vi "LogError.vi"(8 "error in (no error)":errorcluster, 10 "No Error":bool, 11 "Error Message":string) -> (0 "error out":errorcluster)   [LabVIEW 2017, in "Cls_AggHandler.xnode"]
uses:
  <vilib>/Utility/AggHandler/Cls_AggHandler.xnode
panel:
  out "Array":string[](array[string])
  in  "Clear":bool
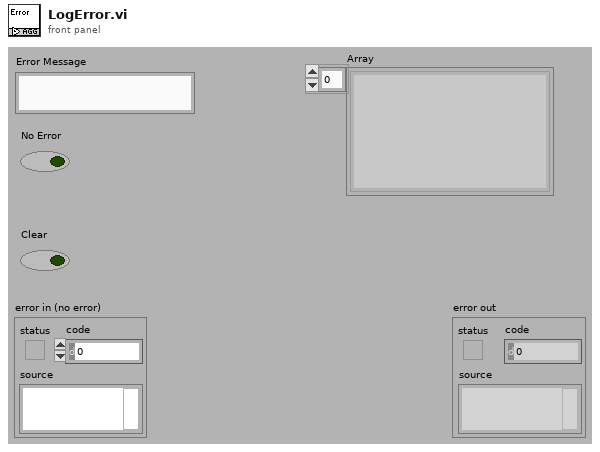
[diagram p1: front panel]
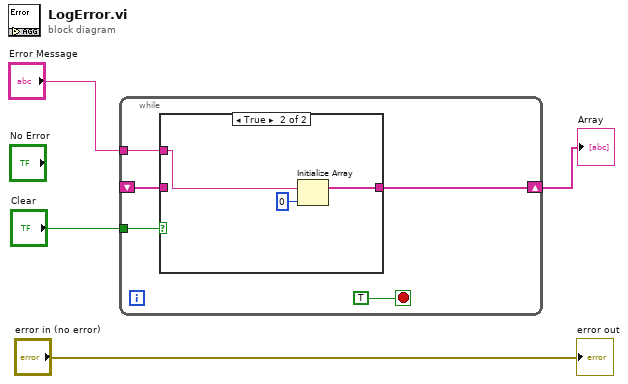
[diagram p0: block diagram]
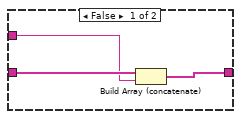
[diagram p2: hidden frame]
diagram:
  n1 = while {
    shift-right: [w6] -> w1
    shift-left: _ -> [w5]
    tunnel: "Clear" -> [w8]
    tunnel: "Error Message" -> [w7]
    stop <- TRUE stop-if-true
    n2 = case shown="True" w8 {
      tunnel: w7 -> [w11 w15]
      tunnel: [w10 w13] -> w6
      tunnel: w5 -> [w12 _]
      frame False {
        n3 = Build Array (concatenate)(w12, w11) -> (w10:string[])
      }
      frame True {
        n4 = Initialize Array(w15, 0 ("dimension size")) -> (w13:string[])
      }
    }
  }
  "Array" <- w1
  "error out" <- "error in (no error)"
